vi "FlexRay_Data_Fold.vi"(10 "FR_Buffer":T1[](array[typedef]), 11 "Fold Data":bool) -> (2 "FR_Buffer out":T1[](array[typedef]))   [LabVIEW 2014]
uses:
  Typedef/TLibFLexRay.ctl
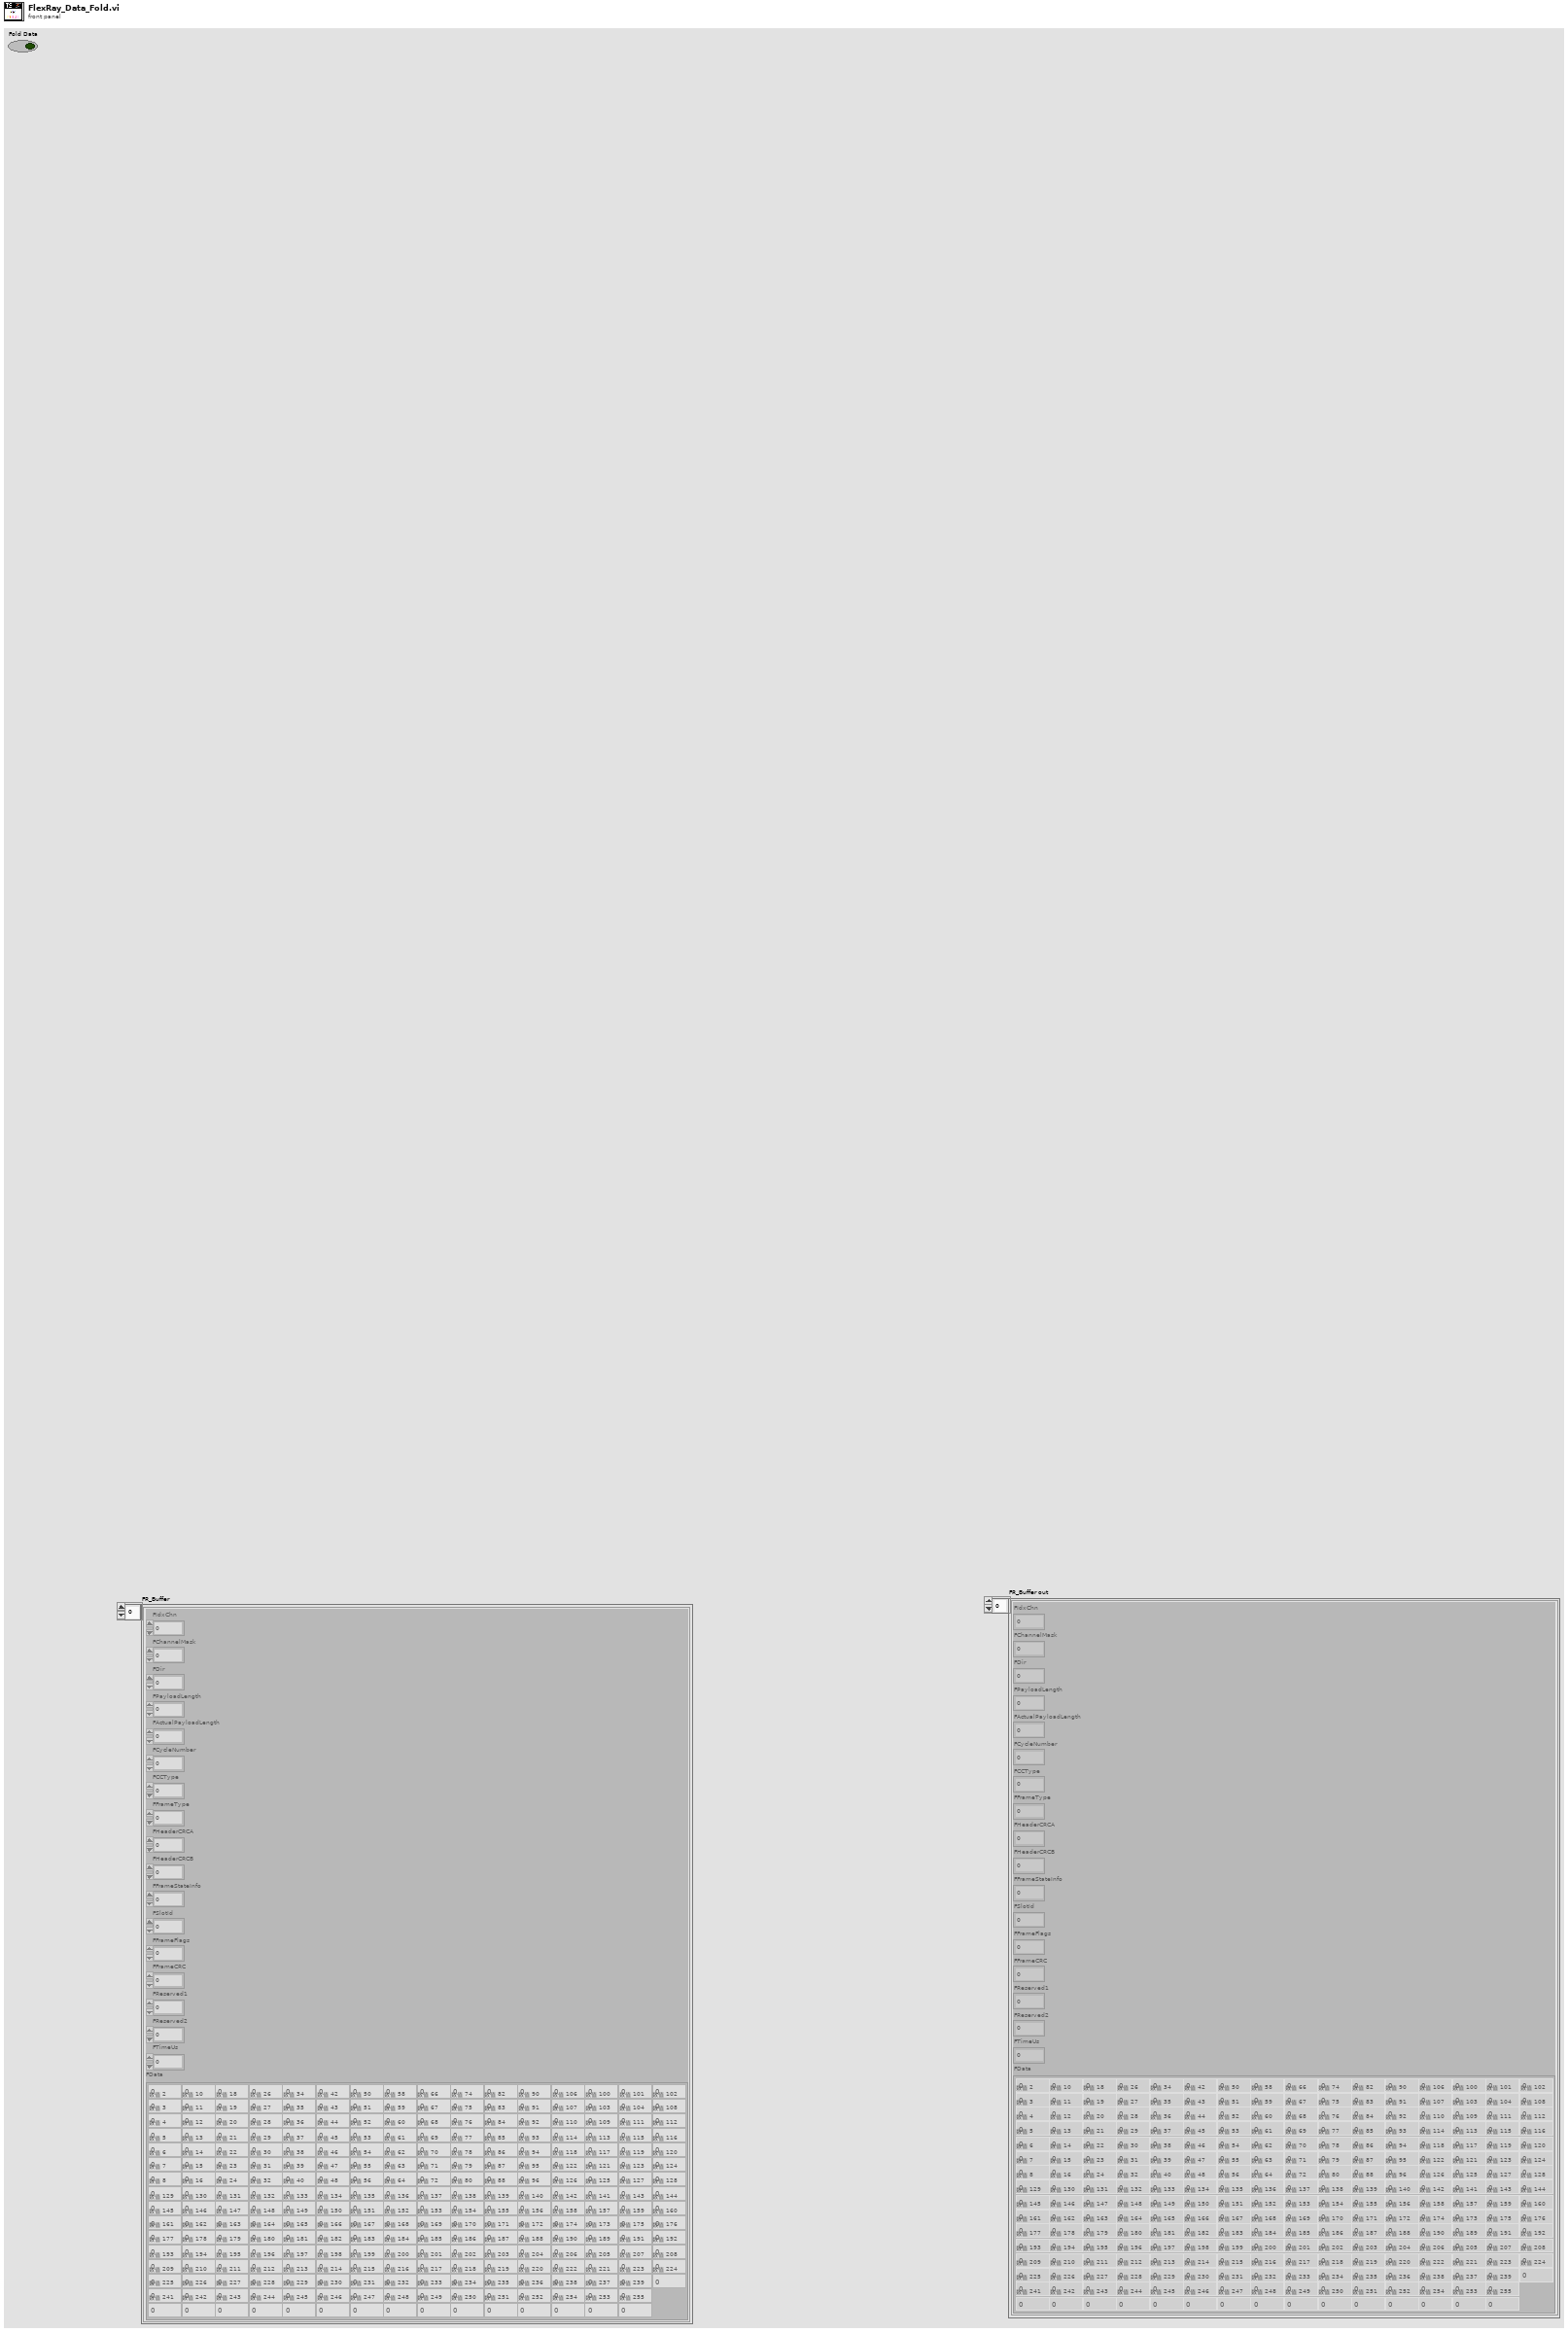
[diagram p1: front panel]
types:
  T1 = typedef "TLibFLexRay.ctl" = cluster{"FIdxChn":u8, "FChannelMask":u8, "FDir":u8, "FPayloadLength":u8, "FActualPayloadLength":u8, "FCycleNumber":u8, "FCCType":u8, "FFrameType":u8, "FHeaderCRCA":u16, "FHeaderCRCB":u16, "FFrameStateInfo":u16, "FSlotId":u16, "FFrameFlags":u32, "FFrameCRC":u32, "FReserved1":u64, "FReserved2":u64, "FTimeUs":u64, "FData":cluster{"数值":u8, "数值 9":u8, "数值 17":u8, "数值 25":u8, "数值 33":u8, "数值 41":u8, "数值 49":u8, "数值 57":u8, "数值 65":u8, "数值 73":u8, "数值 81":u8, "数值 89":u8, "数值 97":u8, "数值 105":u8, "数值 98":u8, "数值 99":u8, "数值 2":u8, "数值 10":u8, "数值 18":u8, "数值 26":u8, "数值 34":u8, "数值 42":u8, "数值 50":u8, "数值 58":u8, "数值 66":u8, "数值 74":u8, "数值 82":u8, "数值 90":u8, "数值 100":u8, "数值 106":u8, "数值 101":u8, "数值 102":u8, "数值 3":u8, "数值 11":u8, "数值 19":u8, "数值 27":u8, "数值 35":u8, "数值 43":u8, "数值 51":u8, "数值 59":u8, "数值 67":u8, "数值 75":u8, "数值 83":u8, "数值 91":u8, "数值 103":u8, "数值 107":u8, "数值 104":u8, "数值 108":u8, "数值 4":u8, "数值 12":u8, "数值 20":u8, "数值 28":u8, "数值 36":u8, "数值 44":u8, "数值 52":u8, "数值 60":u8, "数值 68":u8, "数值 76":u8, "数值 84":u8, "数值 92":u8, "数值 109":u8, "数值 110":u8, "数值 111":u8, "数值 112":u8, "数值 5":u8, "数值 13":u8, "数值 21":u8, "数值 29":u8, "数值 37":u8, "数值 45":u8, "数值 53":u8, "数值 61":u8, "数值 69":u8, "数值 77":u8, "数值 85":u8, "数值 93":u8, "数值 113":u8, "数值 114":u8, "数值 115":u8, "数值 116":u8, "数值 6":u8, "数值 14":u8, "数值 22":u8, "数值 30":u8, "数值 38":u8, "数值 46":u8, "数值 54":u8, "数值 62":u8, "数值 70":u8, "数值 78":u8, "数值 86":u8, "数值 94":u8, "数值 117":u8, "数值 118":u8, "数值 119":u8, "数值 120":u8, "数值 7":u8, "数值 15":u8, "数值 23":u8, "数值 31":u8, "数值 39":u8, "数值 47":u8, "数值 55":u8, "数值 63":u8, "数值 71":u8, "数值 79":u8, "数值 87":u8, "数值 95":u8, "数值 121":u8, "数值 122":u8, "数值 123":u8, "数值 124":u8, "数值 8":u8, "数值 16":u8, "数值 24":u8, "数值 32":u8, "数值 40":u8, "数值 48":u8, "数值 56":u8, "数值 64":u8, "数值 72":u8, "数值 80":u8, "数值 88":u8, "数值 96":u8, "数值 125":u8, "数值 126":u8, "数值 127":u8, "数值 128":u8, "数值 129":u8, "数值 130":u8, "数值 131":u8, "数值 132":u8, "数值 133":u8, "数值 134":u8, "数值 135":u8, "数值 136":u8, "数值 137":u8, "数值 138":u8, "数值 139":u8, "数值 140":u8, "数值 141":u8, "数值 142":u8, "数值 143":u8, "数值 144":u8, "数值 145":u8, "数值 146":u8, "数值 147":u8, "数值 148":u8, "数值 149":u8, "数值 150":u8, "数值 151":u8, "数值 152":u8, "数值 153":u8, "数值 154":u8, "数值 155":u8, "数值 156":u8, "数值 157":u8, "数值 158":u8, "数值 159":u8, "数值 160":u8, "数值 161":u8, "数值 162":u8, "数值 163":u8, "数值 164":u8, "数值 165":u8, "数值 166":u8, "数值 167":u8, "数值 168":u8, "数值 169":u8, "数值 170":u8, "数值 171":u8, "数值 172":u8, "数值 173":u8, "数值 174":u8, "数值 175":u8, "数值 176":u8, "数值 177":u8, "数值 178":u8, "数值 179":u8, "数值 180":u8, "数值 181":u8, "数值 182":u8, "数值 183":u8, "数值 184":u8, "数值 185":u8, "数值 186":u8, "数值 187":u8, "数值 188":u8, "数值 189":u8, "数值 190":u8, "数值 191":u8, "数值 192":u8, "数值 193":u8, "数值 194":u8, "数值 195":u8, "数值 196":u8, "数值 197":u8, "数值 198":u8, "数值 199":u8, "数值 200":u8, "数值 201":u8, "数值 202":u8, "数值 203":u8, "数值 204":u8, "数值 205":u8, "数值 206":u8, "数值 207":u8, "数值 208":u8, "数值 209":u8, "数值 210":u8, "数值 211":u8, "数值 212":u8, "数值 213":u8, "数值 214":u8, "数值 215":u8, "数值 216":u8, "数值 217":u8, "数值 218":u8, "数值 219":u8, "数值 220":u8, "数值 221":u8, "数值 222":u8, "数值 223":u8, "数值 224":u8, "数值 225":u8, "数值 226":u8, "数值 227":u8, "数值 228":u8, "数值 229":u8, "数值 230":u8, "数值 231":u8, "数值 232":u8, "数值 233":u8, "数值 234":u8, "数值 235":u8, "数值 236":u8, "数值 237":u8, "数值 238":u8, "数值 239":u8, "数值 241":u8, "数值 242":u8, "数值 243":u8, "数值 244":u8, "数值 245":u8, "数值 246":u8, "数值 247":u8, "数值 248":u8, "数值 249":u8, "数值 250":u8, "数值 251":u8, "数值 252":u8, "数值 253":u8, "数值 254":u8, "数值 255":u8}}
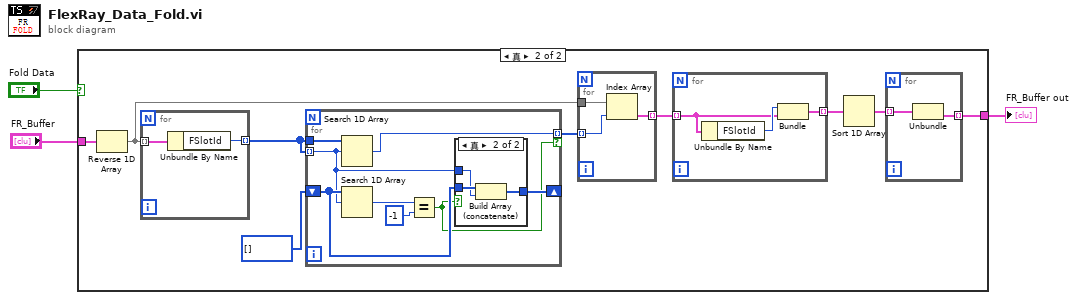
[diagram p0: block diagram]
diagram:
  n1 = case shown="真" "Fold Data" {
    tunnel: [w4 w12] -> w1
    tunnel: "FR_Buffer" -> [w4 w6]
    frame False {
    }
    frame True {
      n2 = Reverse 1D Array(array=w6) -> (reversed array=w5:T1[])
      n3 = for {
        tunnel: w5 -> [w30] mode=indexing
        tunnel: [w29] -> w9 mode=indexing
        n4 = Unbundle By Name(w30) -> ("FSlotId"=w29:u16)
      }
      n5 = for {
        tunnel: w9 -> [w19] mode=indexing
        shift-right: [w24] -> _
        shift-left: u32[] [] -> [w23]
        tunnel: [w18] -> w7 mode=indexing if=w17
        tunnel: w9 -> [w20]
        n6 = Search 1D Array(1D array=w20, element=w19) -> (index of element=w18:i32)  [unwired: 1 in]
        n7 = Search 1D Array(1D array=w23, element=w19) -> (index of element=w21:i32)  [unwired: 1 in]
        n8 = Equal?(x=w21, y=-1) -> (x = y?=w17:bool)
        n9 = case shown="真" w17 {
          tunnel: [w25 w26] -> w24
          tunnel: w23 -> [w25 w28]
          tunnel: w19 -> [_ w27]
          frame False {
          }
          frame True {
            n10 = Build Array (concatenate)(w28, w27) -> (w26:u32[])
          }
        }
      }
      n11 = for {
        tunnel: w5 -> [w16]
        tunnel: w7 -> [w15] mode=indexing
        tunnel: [w14] -> w13 mode=indexing
        n12 = Index Array(array=w16, index=w15) -> (element=w14:T1)
      }
      n13 = for {
        tunnel: w13 -> [w34] mode=indexing
        tunnel: [w33] -> w11 mode=indexing
        n14 = Unbundle By Name(w34) -> ("FSlotId"=w35:u16)
        n15 = Bundle("FSlotId"=w35, "TLibFLexRay"=w34) -> (w33:cluster{"FSlotId":u16, "TLibFLexRay":T1})  [unwired: 1 in]
      }
      n16 = Sort 1D Array(array=w11) -> (sorted array=w10:cluster{"FSlotId":u16, "TLibFLexRay":T1}[])
      n17 = for {
        tunnel: w10 -> [w32] mode=indexing
        tunnel: [w31] -> w12 mode=indexing
        n18 = Unbundle(w32) -> ("TLibFLexRay"=w31:T1)  [unwired: 1 out]
      }
    }
  }
  "FR_Buffer out" <- w1
